vi "ALTS-2015 Status Message Display.vi"(4 "Custom Message?":bool, 6 "Station Message?":bool=TRUE, 7 "Status Message Options":T2, 8 "error in (no error)":errorcluster, 9 "Status Message":refnum<vi>, 10 "Status String IN":string, 11 "Station Enum":T1) -> (0 "error out":errorcluster, 3 "Status String out":string)   [LabVIEW 2013]
uses:
  Controls/ALTS-2015 Status Message Options.ctl
  Controls/ALTS-2015 Station Cluster.ctl
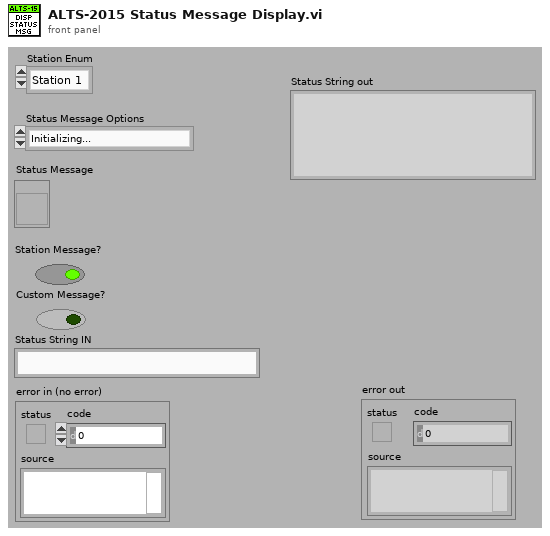
[diagram p1: front panel]
types:
  T1 = typedef "ALTS-2015 Station Cluster.ctl" = enum16{"Station 1", "Station 2", "Station 3", "Station 4"}
  T2 = typedef "ALTS-2015 Status Message Options.ctl" = enum16{"Initializing...", "Enter User Login...", "Valid Serial Number...", "Invalid Serial Number...", "Start Tag Received...", "Stop Tag Received...", "UUT Clamped...", "UUT not Clamped...", "Test Running...", "Test Complete...", "Task is assigned to robot...", "Robot is working on the task...", "Robot is ready for next task...", "Writing Result to DB...", "Idle...", "Exiting..."}
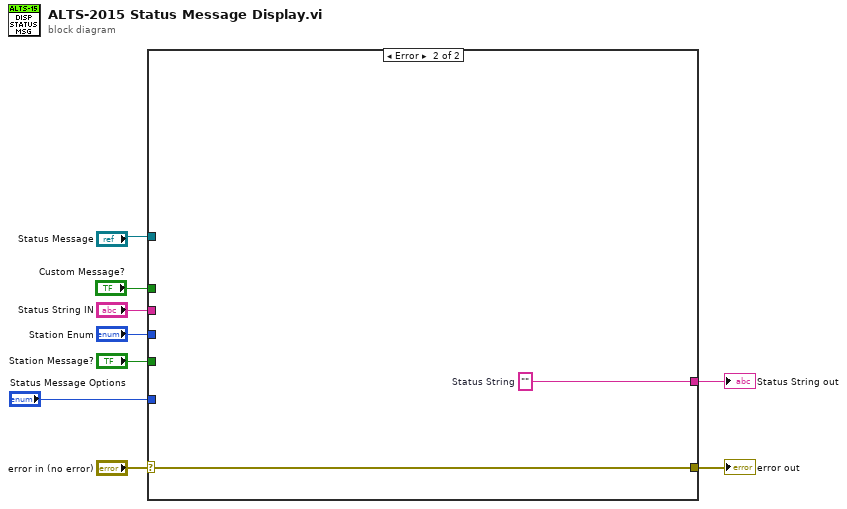
[diagram p0: block diagram]
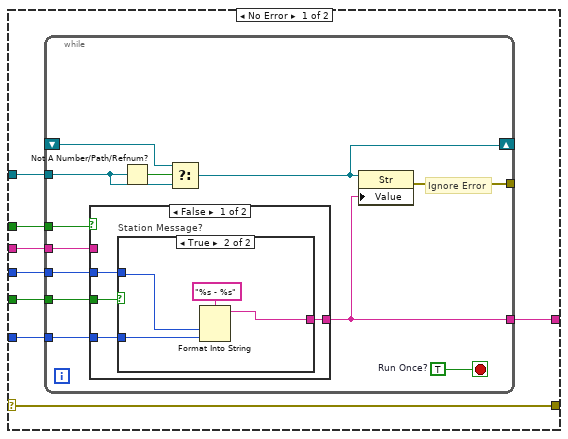
[diagram p2: hidden frame]
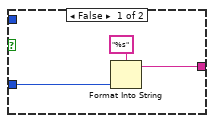
[diagram p3: hidden frame]
diagram:
  n1 = case shown="Error" "error in (no error)" {
    selector: "error in (no error)" -> [w17 w43]
    tunnel: [w17 w43] -> w8
    tunnel: "Station Message?" -> [w16 _]
    tunnel: "Status Message" -> [w15 _]
    tunnel: "Status Message Options" -> [w14 _]
    tunnel: [w13 w42] -> w5
    tunnel: "Station Enum" -> [w12 _]
    tunnel: "Custom Message?" -> [w11 _]
    tunnel: "Status String IN" -> [w10 _]
    frame No Error {
      n2 = while {
        shift-right: [w28] -> _
        shift-left: _ -> [w27]
        tunnel: [w26] -> _
        tunnel: w16 -> [w25]
        tunnel: w15 -> [w24]
        tunnel: w14 -> [w23]
        tunnel: [w22] -> w13
        tunnel: w12 -> [w20]
        tunnel: w11 -> [w19]
        tunnel: w10 -> [w18]
        stop <- w29 stop-if-true
        w29 = TRUE  # Run Once?
        # "Ignore Error"
        n3 = case shown="False" w19 {
          tunnel: w25 -> [w33 _]
          tunnel: w23 -> [w32 _]
          tunnel: [w31 w41] -> w22
          tunnel: w20 -> [w30 _]
          tunnel: w18 -> [_ w41]
          frame False {
            n4 = case "Station Message?" shown="True" w33 {
              tunnel: [w35 w38] -> w31
              tunnel: w32 -> [w34 w37]
              tunnel: w30 -> [_ w39]
              frame False {
                n5 = Format Into String(format string="%s", w34) -> (resulting string=w35:string)  [unwired: 2 in, 1 out]
              }
              frame True {
                n6 = Format Into String(format string="%s - %s", w39, w37) -> (resulting string=w38:string)  [unwired: 2 in, 1 out]
              }
            }
          }
          frame True {
          }
        }
        n7 = Not A Number/Path/Refnum?(number/path/refnum=w24) -> (NaN/Path/Refnum?=w21:bool)
        n8 = Select(t=w27, s=w21, f=w24) -> (s? t:f=w28:refnum<vi>)
        n9 = property on="Property Node" class="Str"(reference=w28, "Value"=w22) -> (error out=w26:errorcluster)  [unwired: 1 in, 1 out]
      }
    }
    frame Error {
      w42 = ""  # Status String
    }
  }
  "error out" <- w8
  "Status String out" <- w5
